vi "AlazarResetTimeStamp.vi"(3 "error in (no error)":errorcluster, 4 "Option":u32(ring) items=["Reset First Time Only", "Reset Always"], 5 "Handle":u64) -> (0 "error out":errorcluster, 1 "Return Code":u32, 2 "Handle":u64)   [LabVIEW 2009]
doc: "Control record timestamp counter resets."
uses:
  ATSApi.dll
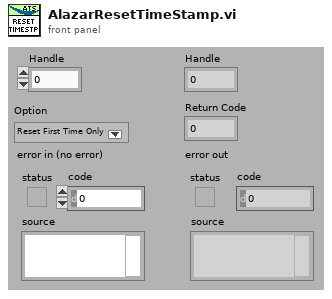
[diagram p1: front panel]
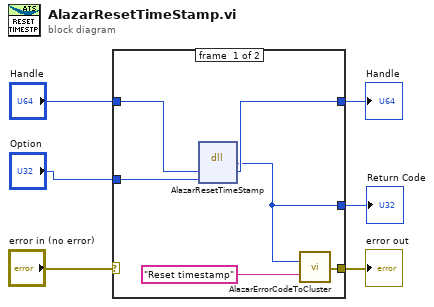
[diagram p0: block diagram]
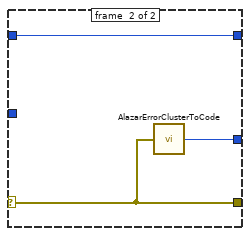
[diagram p2: hidden frame]
diagram:
  n1 = case shown="No Error" "error in (no error)" {
    selector: "error in (no error)" -> [_ w15]
    tunnel: [w9 w15] -> w5
    tunnel: [w8 w14] -> w4
    tunnel: "Handle" -> [w12 w13]
    tunnel: [w11 w13] -> w2
    tunnel: "Option" -> [w10 _]
    frame #0 {
      n2 = dll-call lib="ATSApi.dll" fn="AlazarResetTimeStamp"("handle"=w12, "option"=w10) -> ("return type"=w8:u32, "handle"=w11:u64)  [unwired: 4 in, 2 out]
      n3 = call "AlazarErrorCodeToCluster.vi"("Message"="Reset timestamp", "Error Code"=w8) -> ("error out"=w9:errorcluster)
    }
    frame #1 {
      n4 = call "AlazarErrorClusterToCode.vi"("error in (no error)"=w15) -> ("Error Code"=w14:u32)
    }
  }
  "Handle" <- w2
  "error out" <- w5
  "Return Code" <- w4
